vi "TPM with correction version 10-3-compare-1 scale factor.vi"() -> ()   [LabVIEW 2012]
uses:
  <vilib>/_Imagine Optic/VIs drivers/Data Haso/Wavefront parameters.ctl
  Program Files/Imagine Optic/Casao LabVIEW SDK/Casao/Casao/Loop prefs.ctl
  <vilib>/_Imagine Optic/VIs drivers/Data Haso/DataHaso.ctl
  <vilib>/Utility/file.llb/Read From Spreadsheet File (DBL).vi
  <vilib>/Utility/file.llb/Write To Spreadsheet File (DBL).vi
panel:
  in  "Scale factor":dbl=1.0
  out "output path":path
  out "Model Coefficients (µm) after":sgl[](array[numeric])
  out "Model Coefficients (µm) before":sgl[](array[numeric])
  in  "stop":bool
  out "Slice now":dbl
  in  "Iteration #":u16(ring)=1 items=["1"=1, "2"=2, "3"=3, "4"=4, "5"=5]
  in  "AoExp Time":dbl(ring)=0.5 items=["0.2s"=0.2, "0.5s"=0.5, "1.0s"=1.0, "1.5s"=1.5]
  out "after correction":T1
  in  "Filter y tilt":bool=TRUE
  in  "Filter x tilt":bool=TRUE
  in  "Curvature filter":bool=TRUE
  out "PV":dbl
  out "RMS":dbl
  in  "Matrix path":path=path "C:/Documents and Settings/User/Desktop/zw/20160128 1um bead command matrix.aomc"
  in  "Offset path":path=path "C:/Documents and Settings/User/Desktop/zw/2016-02-09 system resolution/100nm bead correction.dat"
  out "Camera image":u32[][](graph)
  out "RMS":dbl
  out "PV":dbl
  out "before correction":T1
  in  "Curvature filter":bool=TRUE
  in  "Filter y tilt":bool=TRUE
  in  "Filter x tilt":bool=TRUE
  out "after correction":dbl[][](graph) caption="Wavefront"
  out "before correction":dbl[][](graph) caption="Wavefront"
  in  "ImExp Time (s)":dbl(ring)=0.5 items=["0.2"=0.2, "0.5"=0.5, "1.0"=1.0, "4.0"=4.0, "8.0"=8.0]
  in  "Step size(um)":dbl
  in  "Laser Power%(0-100)":dbl=10.0
  in  "Slices #":dbl=1.0
  in  "Average Frame #":dbl=10.0
  in  "Correction":bool
  # "OFF"
  # "ON"
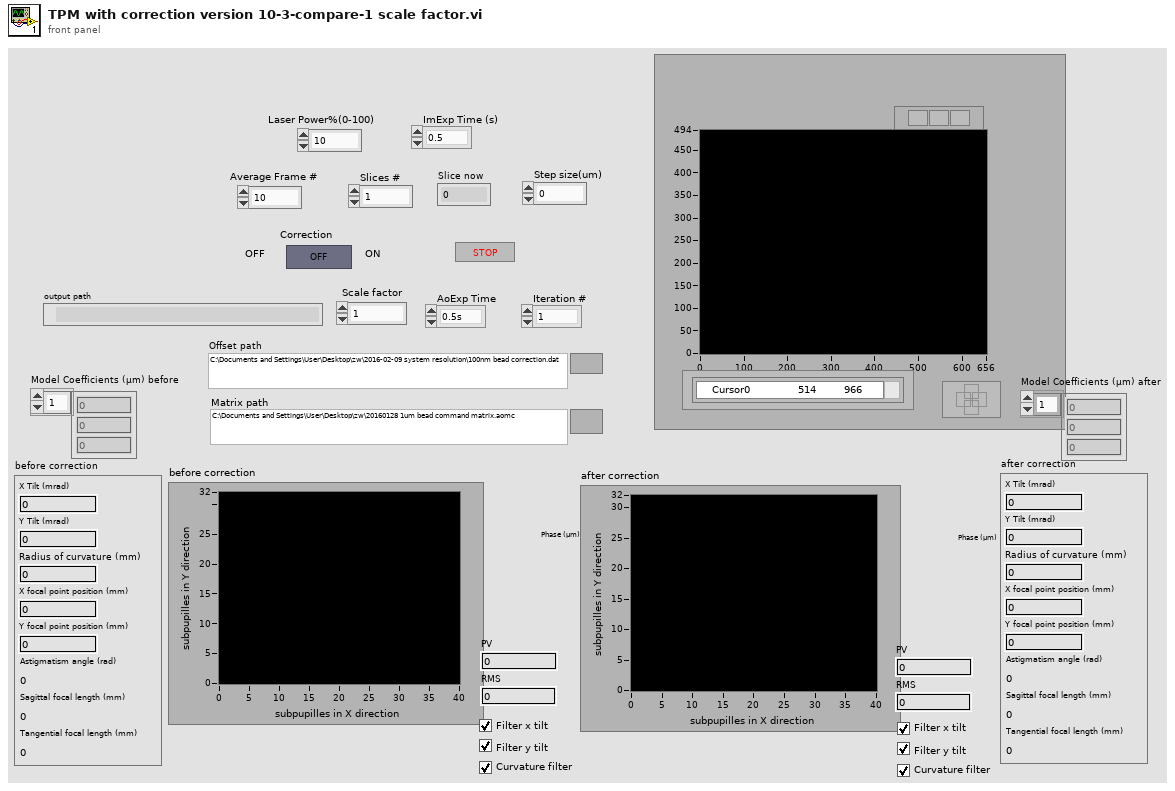
[diagram p1: front panel]
types:
  T1 = typedef "Wavefront parameters.ctl" = cluster{"X Tilt (mrad)":sgl, "Y Tilt (mrad)":sgl, "Radius of curvature (mm)":sgl, "X focal point position (mm)":sgl, "Y focal point position (mm)":sgl, "Astigmatism angle (rad)":sgl, "Sagittal focal length (mm)":sgl, "Tangential focal length (mm)":sgl}
  T2 = typedef "Loop prefs.ctl" = cluster{"Filter tilt on measurement (closed loop)":bool, "Correction gain (closed loop)":sgl, "Limit of subapertures off in CGP (%)":sgl, "Limit of saturated actuators (%)":sgl}
  T3 = cluster{"Filtre tilt X":bool, "Filtre tilt Y":bool, "Filtre courbure":bool}
  T4 = typedef "DataHaso.ctl" = i32
  T5 = cluster{"Measurement":T4, "Target":T4, "Manual target":T4}
  T6 = cluster{"Target for tilt":T4, "Target for focus":T4, "Target for all other aberrations":T4}
  T7 = typedef "Camera.ctl" = i32
  T8 = typedef "PhaseModul.ctl" = i32
  T9 = typedef "Haso.ctl" = i32
  T10 = typedef "Casao.ctl" = i32
  T11 = typedef "Image Compat.ctl" = cluster{"Signed/unsigned":bool, "Number of bits":T12, "Internal object id":i32, "Internal data id":i32}
  T12 = typedef "Data alignment enum.ctl" = enum16{"8", "16", "32"}
  T13 = typedef "Reconstruction prefs.ctl" = cluster{"Reconstruction type":enum16{"Modal", "Zonal"}, "Polynomial type":enum16{"Zernike", "Legendre"}, "Modal reconstruction prefs":T14, "Zonal reconstruction prefs":T17}
  T14 = typedef "Modal reconstruction prefs.ctl" = cluster{"Number of coefficients":u32, "Filtered coefficients":u32[], "RMS Zernike normalization":bool, "Matrix inversion method":u16, "Add zonal residual to modal fit ":bool, "Detection prefs":T15}
  T15 = typedef "PupilDetectionPrefs.ctl" = cluster{"Automatic pupil detection":bool, "Central occultation pupil":bool, "Semi-automatic pupil detection (find radius)":bool, "Semi-automatic pupil detection (find center)":bool, "Automatic pupil detection mode":enum16{"Contained", "Containing"}, "Start coordinates":cluster{"Pupil center (Zernike)":T16, "Pupil radius (Zernike)":sgl, "Pupil center (Legendre)":T16, "Pupil halfsize (Legendre)":T16}}
  T16 = typedef "Point2Df.ctl" = cluster{"X":sgl, "Y":sgl}
  T17 = typedef "Zonal reconstruction prefs.ctl" = cluster{"Number of weak iterations":u16, "Number of max iterations":u32, "Residual limit":sgl}
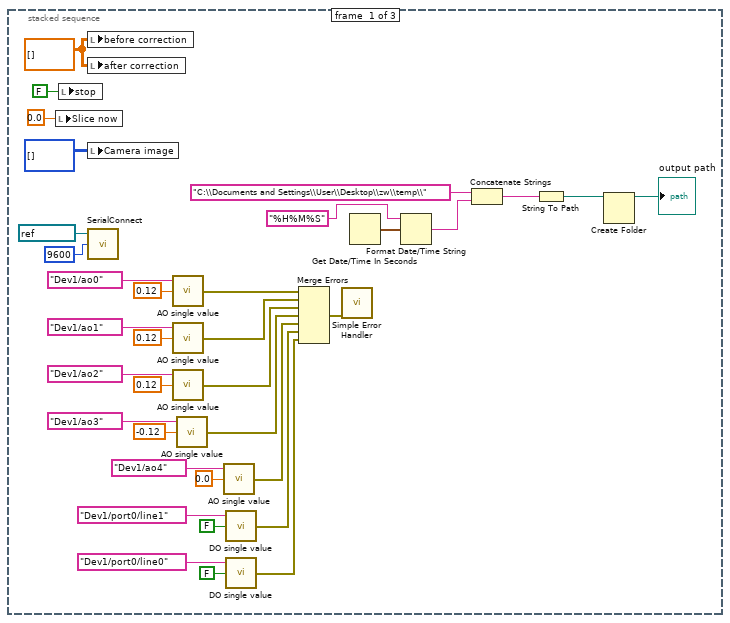
[diagram p2: hidden frame]
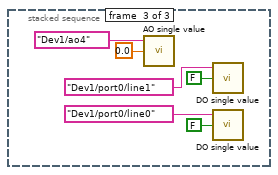
[diagram p11: hidden frame]
diagram:
  n1 = stacked-sequence {
    frame #0 {
      w34 = dbl[][] [] ("before correction")
      n2 = local write "Slice now"(0.0 ("Slice now")) -> ()
      n3 = local write "stop"(FALSE ("stop")) -> ()
      n4 = local write "before correction"(w34) -> ()
      n5 = local write "after correction"(w34) -> ()
      n6 = local write "Camera image"(u32[][] [] ("Camera image")) -> ()
      n7 = call "SerialConnect.vi"("baud rate (9600)"=u32 9600, "VISA resource name"=refnum<visa-resource-name> "COM1") -> ()  [unwired: 1 in, 3 out]
      n8 = call "AO single value.vi"("data"=0.12, "physical channels"=tag "Dev1/ao0") -> ("error out"=w17:errorcluster)  [unwired: 1 in]
      n9 = call "AO single value.vi"("data"=0.12, "physical channels"=tag "Dev1/ao1") -> ("error out"=w16:errorcluster)  [unwired: 1 in]
      n10 = call "AO single value.vi"("data"=0.12, "physical channels"=tag "Dev1/ao2") -> ("error out"=w15:errorcluster)  [unwired: 1 in]
      n11 = call "AO single value.vi"("data"=-0.12, "physical channels"=tag "Dev1/ao3") -> ("error out"=w14:errorcluster)  [unwired: 1 in]
      n12 = call "AO single value.vi"("data"=0.0, "physical channels"=tag "Dev1/ao4") -> ("error out"=w13:errorcluster)  [unwired: 1 in]
      n13 = call "DO single value.vi"("data"=FALSE, "lines"=tag "Dev1/port0/line1") -> ("error out"=w12:errorcluster)  [unwired: 1 in]
      n14 = call "DO single value.vi"("data"=FALSE, "lines"=tag "Dev1/port0/line0") -> ("error out"=w10:errorcluster)  [unwired: 1 in]
      n15 = Merge Errors(w17, w16, w15, w14, w13, w12, w10) -> (w11:errorcluster)
      n16 = call <vilib>:"Simple Error Handler.vi"("error in (no error)"=w11) -> ()  [unwired: 4 in, 5 out]
      n17 = Get Date/Time In Seconds() -> (seconds since 1Jan1904=w7:timestamp)
      n18 = Format Date/Time String(time format string (%c)="%H%M%S", seconds (now)=w7) -> (date/time string=w4:string)  [unwired: 1 in]
      n19 = Concatenate Strings("C:\\Documents and Settings\\User\\Desktop\\zw\\temp\\" ("string"), w4) -> (w3:string)
      n20 = String To Path(string=w3) -> (path=w2:path)
      n21 = Create Folder(path (use dialog)=w2) -> (created path=→"output path":path)  [unwired: 2 in, 2 out]
    }
    frame #1 {
      n22 = case shown="False" "Correction" {
        frame False {
          n23 = flat-sequence {
            frame #0 {
              n24 = call "AO single value.vi"("data"=-5.0, "physical channels"=tag "Dev1/ao5") -> ()  [unwired: 1 in, 1 out]
              n25 = call "DO single value.vi"("data"=TRUE, "lines"=tag "Dev1/port0/line1") -> ()  [unwired: 1 in, 1 out]
              n26 = call "DO single value.vi"("data"=FALSE, "lines"=tag "Dev1/port0/line0") -> ()  [unwired: 1 in, 1 out]
            }
            frame #1 {
              n27 = for {
                N: "Slices #" -> [_]
                i -> [w47]
                n28 = local read "stop"() -> (w45:bool)
                n29 = Not(x=w45) -> (.not. x?=w44:bool)
                n30 = Increment(x=w47) -> (x+1=w46:i32)
                n31 = case shown="True" w44 {
                  tunnel: w46 -> [_ w48]
                  frame False {
                  }
                  frame True {
                    n32 = flat-sequence {
                      frame #0 {
                        n33 = for {
                          N: "Average Frame #" -> [_]
                          n34 = local read "stop"() -> (w50:bool)
                          n35 = Not(x=w50) -> (.not. x?=w51:bool)
                          n36 = case shown="True" w51 {
                            frame False {
                            }
                            frame True {
                              n37 = flat-sequence {
                                tunnel: [w53] -> w52
                                tunnel: w52 -> [w75]
                                frame #0 {
                                n38 = local read "Laser Power%(0-100)"() -> (w64:dbl)
                                n39 = local read "ImExp Time (s)"() -> (w63:dbl)
                                n40 = call "waveform gen.vi"("Boolean"=TRUE, "Exposure Time (s)"=w63, "Laser Power%(0-100)"=w64) -> ("waveform"=w61:waveform(dbl)[])
                                n41 = Index Array(array=w61, index=4) -> (element=w62:waveform(dbl))
                                n42 = call "AO triggle.vi"("physical channels"=tag "Dev1/ao0:4", "data"=w61, "waveform"=w62, "trig source"=tag "/Dev1/PFI1") -> ("task out"=w58:refnum<k21>, "error out"=w55:errorcluster)  [unwired: 1 in]
                                n43 = call "DO single value.vi"("error in"=w55, "data"=TRUE, "lines"=tag "Dev1/port0/line0") -> ("error out"=w54:errorcluster)
                                n44 = while {
                                tunnel: [w73] -> w67
                                tunnel: [w72] -> w66
                                tunnel: w58 -> [w70]
                                tunnel: w54 -> [w69]
                                stop <- w71 stop-if-true
                                n45 = call <vilib>:"DAQmx Is Task Done.vi"("task/channels in"=w70, "error in"=w69) -> ("task out"=w73:refnum<k21>, "task done?"=w71:bool, "error out"=w72:errorcluster)  [unwired: 11 in]
                                }
                                n46 = call <vilib>:"DAQmx Clear Task.vi"("task in"=w67, "error in"=w66) -> ("error out"=w53:errorcluster)  [unwired: 13 in]
                                }
                                frame #1 {
                                n47 = call "DO single value.vi"("error in"=w75, "data"=FALSE, "lines"=tag "Dev1/port0/line0") -> ("error out"=w74:errorcluster)
                                n48 = call "AO single value.vi"("error in"=w74, "data"=0.0, "physical channels"=tag "Dev1/ao4") -> ()  [unwired: 1 out]
                                }
                              }
                            }
                          }
                        }
                      }
                      frame #1 {
                        n49 = local read "Step size(um)"() -> (w80:dbl)
                        n50 = Multiply(x=w80, y=10.0) -> (x*y=w82:dbl)
                        n51 = Number To Decimal String(number=w82) -> (decimal integer string=w85:string)  [unwired: 1 in]
                        n52 = Concatenate Strings("movrel z=", w85) -> (w84:string)
                        n53 = call "WriteCmd.vi"("Command"=w84, "VISA resource name"=refnum<visa-resource-name> "COM1") -> ()  [unwired: 1 in, 1 out]
                      }
                      frame #2 {
                        n54 = Wait (ms)(milliseconds to wait=u32 100) -> ()  [unwired: 1 out]
                      }
                    }
                    n55 = local write "Slice now"(w48) -> ()
                  }
                }
              }
            }
            frame #2 {
            }
          }
        }
        frame True {
          n56 = flat-sequence {
            tunnel: [w103] -> w95
            tunnel: [w105] -> w94
            tunnel: [w104] -> w93
            tunnel: [w103] -> w92
            tunnel: [w102] -> w91
            tunnel: [w101] -> w89
            tunnel: [w96] -> w88
            tunnel: w95 -> [w122]
            tunnel: w94 -> [w121]
            tunnel: w93 -> [w120]
            tunnel: w92 -> [w116]
            tunnel: w91 -> [w114]
            tunnel: [w119] -> w90
            tunnel: w89 -> [w118]
            tunnel: w88 -> [w112]
            tunnel: w90 -> [w646]
            frame #0 {
              n57 = call "AO single value.vi"("data"=0.0, "physical channels"=tag "Dev1/ao4") -> ()  [unwired: 1 in, 1 out]
              n58 = local read "AoExp Time"() -> (w106:dbl)
              n59 = call-poly <vilib>:"Read From Spreadsheet File.vi"("format (%.3f)"="%.8f", "file path (dialog if empty)"="Offset path") -> ("first row"=w96:dbl[])  [unwired: 5 in, 4 out]
              n60 = call "DO single value.vi"("data"=TRUE, "lines"=tag "Dev1/port0/line1") -> ()  [unwired: 1 in, 1 out]
              n61 = call "DO single value.vi"("data"=FALSE, "lines"=tag "Dev1/port0/line0") -> ()  [unwired: 1 in, 1 out]
              n62 = call "AO init.vi"("Exposure duration specified (s)"=w106, "Commands in"=w96, "Matrix path"="Matrix path") -> ("error out"=w103:errorcluster, "Camera"=w105:T7, "Mirror"=w101:T8, "Haso"=w104:T9, "Casao"=w102:T10)  [unwired: 3 in, 1 out]
            }
            frame #1 {
              n63 = local read "Slices #"() -> (w123:dbl)
              n64 = call "Casao Set Preferences.vi"("error in (no error)"=w116, "Loop preferences"=T2 {"Filter tilt on measurement (closed loop)"=FALSE, "Correction gain (closed loop)"=0.75, "Limit of subapertures off in CGP (%)"=0.0, "Limit of saturated actuators (%)"=0.0}, "Casao"=w114) -> ("error out"=w115:errorcluster, "Casao (dup)"=w113:T10)  [unwired: 3 in]
              n65 = for {
                N: w123 -> [_]
                tunnel: w122 -> [w139]
                tunnel: w121 -> [w138]
                tunnel: w120 -> [w137]
                tunnel: w115 -> [w125]
                tunnel: [w136] -> w119
                tunnel: w118 -> [w127]
                tunnel: w113 -> [w135]
                tunnel: w112 -> [w128]
                i -> [w131]
                n66 = local read "stop"() -> (w133:bool)
                n67 = call "PhaseModul apply command.vi"("error in (no error)"=w125, "Commands in"=w128, "Mirror"=w127) -> ("error out"=w124:errorcluster, "Mirror (dup)"=w126:T8)  [unwired: 2 in, 1 out]
                n68 = Increment(x=w131) -> (x+1=w134:i32)
                n69 = local write "Slice now"(w134) -> ()
                n70 = Not(x=w133) -> (.not. x?=w132:bool)
                n71 = case shown="True" w132 {
                  tunnel: w139 -> [_ w174]
                  tunnel: w138 -> [_ w173]
                  tunnel: w137 -> [_ w172]
                  tunnel: w124 -> [_ w171]
                  tunnel: [w140 w168] -> w136
                  tunnel: w126 -> [_ w170]
                  tunnel: w135 -> [w140 w169]
                  frame False {
                  }
                  frame True {
                    n72 = flat-sequence {
                      tunnel: w169 -> [w179]
                      tunnel: w170 -> [w180]
                      tunnel: w171 -> [w181]
                      tunnel: w172 -> [w182]
                      tunnel: w173 -> [w183]
                      tunnel: w174 -> [w184]
                      tunnel: [w184] -> w146
                      tunnel: [w183] -> w145
                      tunnel: [w182] -> w144
                      tunnel: [w181] -> w143
                      tunnel: [w180] -> w142
                      tunnel: [w179] -> w141
                      tunnel: [w218] -> w167
                      tunnel: [w217] -> w166
                      tunnel: [w216] -> w165
                      tunnel: [w211] -> w164
                      tunnel: [w212] -> w163
                      tunnel: [w213] -> w162
                      tunnel: w146 -> [w218]
                      tunnel: w145 -> [w217]
                      tunnel: w144 -> [w216]
                      tunnel: w143 -> [w212]
                      tunnel: w142 -> [w213]
                      tunnel: w141 -> [w211]
                      tunnel: w167 -> [w260]
                      tunnel: w166 -> [w259]
                      tunnel: w165 -> [w258]
                      tunnel: w164 -> [w257]
                      tunnel: w163 -> [w256]
                      tunnel: [w236] -> w161
                      tunnel: [w235] -> w160
                      tunnel: [w231] -> w159
                      tunnel: [w229] -> w158
                      tunnel: [w227] -> w157
                      tunnel: w162 -> [w222]
                      tunnel: [w221] -> w156
                      tunnel: [w219] -> w155
                      tunnel: w161 -> [w402]
                      tunnel: w160 -> [w401]
                      tunnel: w159 -> [w399]
                      tunnel: w158 -> [w398]
                      tunnel: w157 -> [w397]
                      tunnel: [w396] -> w154
                      tunnel: w156 -> [w395]
                      tunnel: [w394] -> w153
                      tunnel: [w393] -> w152
                      tunnel: [w392] -> w151
                      tunnel: [w391] -> w150
                      tunnel: [w390] -> w149
                      tunnel: w155 -> [w389]
                      tunnel: [w389] -> w148
                      tunnel: w154 -> [w609]
                      tunnel: [w609] -> w147
                      tunnel: w153 -> [w599]
                      tunnel: w152 -> [w598]
                      tunnel: w151 -> [w597]
                      tunnel: w150 -> [w587]
                      tunnel: w149 -> [w588]
                      tunnel: w148 -> [w586]
                      tunnel: w147 -> [w610]
                      tunnel: [w610] -> w168
                      frame #0 {
                        n73 = Wait (ms)(milliseconds to wait=u32 100) -> ()  [unwired: 1 out]
                        n74 = local read "Average Frame #"() -> (w178:dbl)
                        n75 = call "AO single value.vi"("data"=-5.0, "physical channels"=tag "Dev1/ao5") -> ()  [unwired: 1 in, 1 out]
                        n76 = for {
                          N: w178 -> [_]
                          n77 = local read "stop"() -> (w185:bool)
                          n78 = Not(x=w185) -> (.not. x?=w186:bool)
                          n79 = case shown="True" w186 {
                            frame False {
                            }
                            frame True {
                              n80 = flat-sequence {
                                frame #0 {
                                n81 = local read "Laser Power%(0-100)"() -> (w197:dbl)
                                n82 = local read "ImExp Time (s)"() -> (w196:dbl)
                                n83 = call "waveform gen.vi"("Boolean"=TRUE, "Exposure Time (s)"=w196, "Laser Power%(0-100)"=w197) -> ("waveform"=w194:waveform(dbl)[])
                                n84 = Index Array(array=w194, index=4) -> (element=w195:waveform(dbl))
                                n85 = call "AO triggle.vi"("physical channels"=tag "Dev1/ao0:4", "data"=w194, "waveform"=w195, "trig source"=tag "/Dev1/PFI0") -> ("task out"=w191:refnum<k21>, "error out"=w188:errorcluster)  [unwired: 1 in]
                                n86 = call "DO single value.vi"("error in"=w188, "data"=TRUE, "lines"=tag "Dev1/port0/line0") -> ("error out"=w187:errorcluster)
                                n87 = while {
                                tunnel: [w206] -> w200
                                tunnel: [w205] -> w199
                                tunnel: w191 -> [w203]
                                tunnel: w187 -> [w202]
                                stop <- w204 stop-if-true
                                n88 = call <vilib>:"DAQmx Is Task Done.vi"("task/channels in"=w203, "error in"=w202) -> ("task out"=w206:refnum<k21>, "task done?"=w204:bool, "error out"=w205:errorcluster)  [unwired: 11 in]
                                }
                                n89 = call <vilib>:"DAQmx Clear Task.vi"("task in"=w200, "error in"=w199) -> ()  [unwired: 13 in, 1 out]
                                }
                                frame #1 {
                                n90 = call "AO single value.vi"("data"=0.0, "physical channels"=tag "Dev1/ao4") -> ()  [unwired: 1 in, 1 out]
                                n91 = call "DO single value.vi"("data"=FALSE, "lines"=tag "Dev1/port0/line0") -> ()  [unwired: 1 in, 1 out]
                                }
                              }
                            }
                          }
                        }
                      }
                      frame #1 {
                        n92 = call "AO single value.vi"("data"=1.0, "physical channels"=tag "Dev1/ao5") -> ()  [unwired: 1 in, 1 out]
                      }
                      frame #2 {
                        n93 = flat-sequence {
                          tunnel: [w269] -> w255
                          tunnel: [w268] -> w254
                          tunnel: [w267] -> w253
                          tunnel: [w266] -> w252
                          tunnel: [w265] -> w251
                          tunnel: w258 -> [w267]
                          tunnel: w259 -> [w268]
                          tunnel: w260 -> [w269]
                          tunnel: [w264] -> w250
                          tunnel: w257 -> [w264]
                          tunnel: [w263] -> w249
                          tunnel: w256 -> [w263]
                          tunnel: [w262] -> w223
                          tunnel: w222 -> [w262]
                          tunnel: w255 -> [w285]
                          tunnel: w254 -> [w286]
                          tunnel: w253 -> [w287]
                          tunnel: [w287] -> w248
                          tunnel: [w284] -> w247
                          tunnel: [w283] -> w246
                          tunnel: [w282] -> w245
                          tunnel: w252 -> [w282]
                          tunnel: [w281] -> w244
                          tunnel: w251 -> [w281]
                          tunnel: [w280] -> w243
                          tunnel: w250 -> [w280]
                          tunnel: [w279] -> w242
                          tunnel: w249 -> [w279]
                          tunnel: [w278] -> w224
                          tunnel: w223 -> [w278]
                          tunnel: w248 -> [w299]
                          tunnel: [w299] -> w239
                          tunnel: [w298] -> w240
                          tunnel: w247 -> [w298]
                          tunnel: [w297] -> w241
                          tunnel: w246 -> [w297]
                          tunnel: w245 -> [w292]
                          tunnel: w244 -> [w291]
                          tunnel: [w290] -> w238
                          tunnel: w243 -> [w290]
                          tunnel: [w289] -> w237
                          tunnel: w242 -> [w289]
                          tunnel: [w288] -> w225
                          tunnel: w224 -> [w288]
                          tunnel: w241 -> [w381]
                          tunnel: w240 -> [w341]
                          tunnel: w239 -> [w342]
                          tunnel: w238 -> [w367]
                          tunnel: w237 -> [w366]
                          tunnel: [w345] -> w234
                          tunnel: [w344] -> w233
                          tunnel: [w343] -> w232
                          tunnel: [w342] -> w230
                          tunnel: [w341] -> w228
                          tunnel: [w340] -> w226
                          tunnel: w225 -> [w339]
                          tunnel: [w339] -> w220
                          tunnel: [w313] -> w219
                          tunnel: [w387] -> w235
                          tunnel: [w388] -> w236
                          tunnel: w234 -> [w388]
                          tunnel: w233 -> [w387]
                          tunnel: w232 -> [w386]
                          tunnel: [w385] -> w231
                          tunnel: w230 -> [w385]
                          tunnel: [w384] -> w229
                          tunnel: w228 -> [w384]
                          tunnel: [w383] -> w227
                          tunnel: w226 -> [w383]
                          tunnel: [w382] -> w221
                          tunnel: w220 -> [w382]
                          frame #0 {
                            n94 = local read "Laser Power%(0-100)"() -> (w275:dbl)
                            n95 = local read "AoExp Time"() -> (w274:dbl)
                            n96 = local read "Scale factor"() -> (w261:dbl)
                            n97 = call "waveform gen_scale factor.vi"("Scale factor"=w261, "Boolean"=FALSE, "Exposure Time (s)"=w274, "Laser Power%(0-100)"=w275) -> ("waveform"=w273:waveform(dbl)[])
                            n98 = Index Array(array=w273, index=4) -> (element=w272:waveform(dbl))
                            n99 = call "AO triggle.vi"("physical channels"=tag "Dev1/ao0:4", "data"=w273, "waveform"=w272, "trig source"=tag "/Dev1/PFI1") -> ("task out"=w266:refnum<k21>, "error out"=w265:errorcluster)  [unwired: 1 in]
                          }
                          frame #1 {
                            n100 = call <vilib>:"Camera Start.vi"("error in (no error)"=w285, "camera"=w286) -> ("error out"=w283:errorcluster, "camera (dup)"=w284:T7)  [unwired: 4 in]
                          }
                          frame #2 {
                            n101 = while {
                              tunnel: [w304] -> w294
                              tunnel: [w303] -> w293
                              tunnel: w292 -> [w301]
                              tunnel: w291 -> [w300]
                              stop <- w302 stop-if-true
                              n102 = call <vilib>:"DAQmx Is Task Done.vi"("task/channels in"=w301, "error in"=w300) -> ("task out"=w304:refnum<k21>, "task done?"=w302:bool, "error out"=w303:errorcluster)  [unwired: 11 in]
                            }
                            n103 = call "DO single value.vi"("data"=TRUE, "lines"=tag "Dev1/port0/line0") -> ()  [unwired: 1 in, 1 out]
                            n104 = call <vilib>:"DAQmx Clear Task.vi"("task in"=w294, "error in"=w293) -> ()  [unwired: 13 in, 1 out]
                          }
                          frame #3 {
                            n105 = call <vilib>:"Camera Get image.vi"("error in (no error)"=w381, "camera"=w341) -> ("error out"=w363:errorcluster, "Image"=w364:T11, "camera (dup)"=w365:T7)  [unwired: 3 in]
                            n106 = call <vilib>:"Camera Stop.vi"("error in (no error)"=w363, "camera"=w365) -> ()  [unwired: 4 in, 2 out]
                            n107 = call "Image get data.vi"("error in (no error)"=w363, "Image Compat"=w364) -> ("error out"=w353:errorcluster, "Array"=w362:u32[][], "Image Compat (dup)"=w352:T11)  [unwired: 3 in]
                            n108 = call "AO single value.vi"("data"=0.0, "physical channels"=tag "Dev1/ao4") -> ()  [unwired: 1 in, 1 out]
                            n109 = local write "Camera image"(w362) -> ()
                            n110 = call <vilib>:"Haso compute slopes.vi"("error in (no error)"=w353, "Image Compat"=w352, "Haso"=w342) -> ("error out"=w311:errorcluster, "Data Haso"=w315:T4)  [unwired: 1 in, 2 out]
                            n111 = call "DO single value.vi"("data"=FALSE, "lines"=tag "Dev1/port0/line0") -> ()  [unwired: 1 in, 1 out]
                            n112 = call "DataHaso ctor copie.vi"("error in (no error)"=w311, "DataHaso"=w315) -> ("error out"=w310:errorcluster, "new DataHaso"=w313:T4, "DataHaso (dup)"=w312:T4)  [unwired: 3 in]
                            n113 = call "DataHaso get reconstruction prefs.vi"("error in (no error)"=w310, "Data Haso"=w312) -> ("error out"=w326:errorcluster, "Reconstruction Preferences"=w322:T13, "Data Haso (dup)"=w325:T4)  [unwired: 3 in]
                            n114 = Bundle By Name(cluster=w322, "Reconstruction type"=enum16{"Modal", "Zonal"}."Modal", "Polynomial type"=enum16{"Zernike", "Legendre"}."Zernike", "Modal reconstruction prefs.Number of coefficients"=u32 32) -> (w321:T13)
                            n115 = call <vilib>:"DataHaso set reconstruction prefs.vi"("error in (no error)"=w326, "Reconstruction Preferences"=w321, "Data Haso"=w325) -> ("error out"=w323:errorcluster, "Data Haso (dup)"=w324:T4)  [unwired: 3 in]
                            n116 = call "DataHaso get modal coefficients.vi"("error in (no error)"=w323, "Data Haso"=w324) -> ("error out"=w316:errorcluster, "Coefficients (µm)"=w327:sgl[], "Data Haso (dup)"=w317:T4)  [unwired: 3 in]
                            "Model Coefficients (µm) before" <- w327
                            n117 = Bundle By Name(cluster=T3 {"Filtre tilt X"=FALSE, "Filtre tilt Y"=FALSE, "Filtre courbure"=FALSE} ("Filtre"), "Filtre tilt X"="Filter x tilt", "Filtre tilt Y"="Filter y tilt", "Filtre courbure"="Curvature filter") -> (w347:T3)
                            n118 = call <vilib>:"DataHaso parameters.vi"("error in (no error)"=w316, "Data Haso"=w317) -> ("error out"=w360:errorcluster, "Parameters"=w335:T1, "Data Haso (dup)"=w361:T4)  [unwired: 3 in]
                            "before correction" <- w335
                            n119 = control-ref of="before correction"() -> (w346:refnum<vi>)
                            n120 = Cluster To Array(cluster=w335) -> (array=w336:sgl[])
                            n121 = call "DataHaso filter tilt or curvature.vi"("error in (no error)"=w360, "Filter (default: all true)"=w347, "Data Haso"=w361) -> ("error out"=w358:errorcluster, "Data Haso (dup)"=w359:T4)  [unwired: 3 in]
                            n122 = local read "Slice now"() -> (w329:dbl)
                            n123 = call "DataHaso phase.vi"("error in (no error)"=w358, "Data Haso"=w359) -> ("error out"=w356:errorcluster, "Phase (µm)"=w357:i32, "Data Haso (dup)"=w314:T4)  [unwired: 3 in]
                            n124 = Number To Decimal String(number=w329) -> (decimal integer string=w331:string)  [unwired: 1 in]
                            n125 = call "Formatter Intensity Graph.vi"("error in (no error)"=w356, "Intensity Graph"=w346, "Surface with pupil"=w357) -> ("error out"=w354:errorcluster, "Surface with pupil (dup)"=w355:i32)  [unwired: 2 in, 1 out]
                            n126 = call <vilib>:"Surface with pupil get stats.vi"("error in (no error)"=w354, "Surface Avec Pupille"=w355) -> ("error out"=w340:errorcluster, "PV"=w338:sgl, "RMS"=w337:dbl)  [unwired: 2 in, 1 out]
                            "PV" <- w338
                            "RMS" <- w337
                            n127 = local read "output path"() -> (w307:path)
                            n128 = Concatenate Strings("before_slice", w331, ".dat") -> (w306:string)
                            n129 = Build Path(base path=w307, name or relative path=w306) -> (appended path=w305:path)
                            n130 = Build Array (concatenate)(w338, w337, w336, w327) -> (w334:dbl[])
                            n131 = Merge Errors(w340, w366) -> (w376:errorcluster)
                            n132 = Bundle By Name(cluster=T6 {"Target for tilt"=0, "Target for focus"=0, "Target for all other aberrations"=0} ("References"), "Target for tilt"=w313, "Target for focus"=w313) -> (w379:T6)
                            n133 = call "DataHaso ctor copie.vi"("error in (no error)"=w376, "DataHaso"=w314) -> ("error out"=w378:errorcluster, "new DataHaso"=w377:T4)  [unwired: 3 in, 1 out]
                            n134 = call-poly <vilib>:"Write To Spreadsheet File.vi"("transpose? (no:F)"=TRUE, "format (%.3f)"="%.6f", "1D data"=w334, "file path (dialog if empty)"=w305) -> ()  [unwired: 4 in, 1 out]
                            n135 = call "Casao Compute target.vi"("error in (no error)"=w378, "Targets"=w379, "DataHaso"=w377, "Casao"=w367) -> ("error out"=w374:errorcluster, "DataHaso (dup)"=w343:T4, "Casao (dup)"=w375:T10)  [unwired: 1 out]
                            n136 = Bundle By Name(cluster=T5 {"Measurement"=0, "Target"=0, "Manual target"=0} ("Slopes"), "Measurement"=w314, "Target"=w343) -> (w373:T5)
                            n137 = call "Casao get correction commands.vi"("Casao"=w375, "Slopes"=w373, "error in (no error)"=w374) -> ("Casao (dup)"=w345:T10, "Commands"=w370:sgl[], "error out"=w371:errorcluster)  [unwired: 2 in, 2 out]
                            n138 = call "PhaseModul apply command.vi"("error in (no error)"=w371, "Commands in"=w370, "Mirror"=w339) -> ("error out"=w344:errorcluster)  [unwired: 2 in, 2 out]
                          }
                          frame #4 {
                            n139 = call "DataHaso dtor.vi"("Data Haso"=w386) -> ()  [unwired: 6 in, 1 out]
                          }
                        }
                      }
                      frame #3 {
                        n140 = for {
                          N: "Iteration #" -> [_]
                          tunnel: w402 -> [w431]
                          tunnel: w401 -> [w430]
                          tunnel: w399 -> [w429]
                          tunnel: w398 -> [w428]
                          tunnel: w397 -> [w427]
                          tunnel: [w425] -> w396
                          tunnel: w395 -> [w420]
                          tunnel: [w419] -> w394
                          tunnel: [w417] -> w393
                          tunnel: [w415] -> w392
                          tunnel: [w413] -> w391
                          tunnel: [w410] -> w390
                          tunnel: w389 -> [w409]
                          i -> [w408]
                          n141 = Increment(x=w408) -> (x+1=w407:i32)
                          n142 = flat-sequence {
                            tunnel: [w456] -> w450
                            tunnel: [w457] -> w449
                            tunnel: [w458] -> w448
                            tunnel: [w462] -> w447
                            tunnel: [w461] -> w446
                            tunnel: [w460] -> w445
                            tunnel: [w459] -> w444
                            tunnel: w431 -> [w460]
                            tunnel: w430 -> [w459]
                            tunnel: w429 -> [w458]
                            tunnel: w428 -> [w457]
                            tunnel: w427 -> [w456]
                            tunnel: [w455] -> w421
                            tunnel: w420 -> [w455]
                            tunnel: w407 -> [w453]
                            tunnel: [w452] -> w404
                            tunnel: w450 -> [w479]
                            tunnel: w449 -> [w480]
                            tunnel: w448 -> [w481]
                            tunnel: [w481] -> w443
                            tunnel: [w478] -> w442
                            tunnel: [w477] -> w441
                            tunnel: [w476] -> w440
                            tunnel: w447 -> [w476]
                            tunnel: [w475] -> w439
                            tunnel: w446 -> [w475]
                            tunnel: [w474] -> w438
                            tunnel: w445 -> [w474]
                            tunnel: [w473] -> w437
                            tunnel: w444 -> [w473]
                            tunnel: [w472] -> w422
                            tunnel: w421 -> [w472]
                            tunnel: [w471] -> w405
                            tunnel: w404 -> [w471]
                            tunnel: w443 -> [w494]
                            tunnel: [w494] -> w434
                            tunnel: [w493] -> w435
                            tunnel: w442 -> [w493]
                            tunnel: [w492] -> w436
                            tunnel: w441 -> [w492]
                            tunnel: w440 -> [w487]
                            tunnel: w439 -> [w486]
                            tunnel: [w485] -> w433
                            tunnel: w438 -> [w485]
                            tunnel: [w484] -> w432
                            tunnel: w437 -> [w484]
                            tunnel: [w483] -> w423
                            tunnel: w422 -> [w483]
                            tunnel: [w482] -> w406
                            tunnel: w405 -> [w482]
                            tunnel: w436 -> [w562]
                            tunnel: w435 -> [w563]
                            tunnel: w434 -> [w564]
                            tunnel: w433 -> [w549]
                            tunnel: w432 -> [w548]
                            tunnel: [w528] -> w426
                            tunnel: [w527] -> w424
                            tunnel: w423 -> [w507]
                            tunnel: [w523] -> w418
                            tunnel: [w522] -> w416
                            tunnel: [w521] -> w414
                            tunnel: [w520] -> w412
                            tunnel: [w509] -> w411
                            tunnel: w409 -> [w506]
                            tunnel: w406 -> [w503]
                            tunnel: [w500] -> w403
                            tunnel: w426 -> [w576]
                            tunnel: [w575] -> w425
                            tunnel: w424 -> [w575]
                            tunnel: [w574] -> w419
                            tunnel: w418 -> [w574]
                            tunnel: [w573] -> w417
                            tunnel: w416 -> [w573]
                            tunnel: [w572] -> w415
                            tunnel: w414 -> [w572]
                            tunnel: [w568] -> w413
                            tunnel: w412 -> [w569]
                            tunnel: w411 -> [w571]
                            tunnel: [w571] -> w410
                            tunnel: w403 -> [w570]
                            frame #0 {
                              n143 = local read "Laser Power%(0-100)"() -> (w468:dbl)
                              n144 = local read "AoExp Time"() -> (w467:dbl)
                              n145 = local read "Scale factor"() -> (w451:dbl)
                              n146 = call "waveform gen_scale factor.vi"("Scale factor"=w451, "Boolean"=FALSE, "Exposure Time (s)"=w467, "Laser Power%(0-100)"=w468) -> ("waveform"=w466:waveform(dbl)[])
                              n147 = local read "Iteration #"() -> (w454:u16)
                              n148 = Index Array(array=w466, index=4) -> (element=w465:waveform(dbl))
                              n149 = Less?(x=w454, y=w453) -> (x < y?=w452:bool)
                              n150 = call "AO triggle.vi"("physical channels"=tag "Dev1/ao0:4", "data"=w466, "waveform"=w465, "trig source"=tag "/Dev1/PFI1") -> ("task out"=w462:refnum<k21>, "error out"=w461:errorcluster)  [unwired: 1 in]
                            }
                            frame #1 {
                              n151 = call <vilib>:"Camera Start.vi"("error in (no error)"=w479, "camera"=w480) -> ("error out"=w477:errorcluster, "camera (dup)"=w478:T7)  [unwired: 4 in]
                            }
                            frame #2 {
                              n152 = while {
                                tunnel: [w499] -> w489
                                tunnel: [w498] -> w488
                                tunnel: w487 -> [w496]
                                tunnel: w486 -> [w495]
                                stop <- w497 stop-if-true
                                n153 = call <vilib>:"DAQmx Is Task Done.vi"("task/channels in"=w496, "error in"=w495) -> ("task out"=w499:refnum<k21>, "task done?"=w497:bool, "error out"=w498:errorcluster)  [unwired: 11 in]
                              }
                              n154 = call "DO single value.vi"("data"=TRUE, "lines"=tag "Dev1/port0/line0") -> ()  [unwired: 1 in, 1 out]
                              n155 = call <vilib>:"DAQmx Clear Task.vi"("task in"=w489, "error in"=w488) -> ()  [unwired: 13 in, 1 out]
                            }
                            frame #3 {
                              n156 = call <vilib>:"Camera Get image.vi"("error in (no error)"=w562, "camera"=w563) -> ("error out"=w545:errorcluster, "Image"=w546:T11, "camera (dup)"=w547:T7)  [unwired: 3 in]
                              n157 = call <vilib>:"Camera Stop.vi"("error in (no error)"=w545, "camera"=w547) -> ()  [unwired: 4 in, 2 out]
                              n158 = call "Image get data.vi"("error in (no error)"=w545, "Image Compat"=w546) -> ("error out"=w535:errorcluster, "Array"=w544:u32[][], "Image Compat (dup)"=w534:T11)  [unwired: 3 in]
                              n159 = call "AO single value.vi"("data"=0.0, "physical channels"=tag "Dev1/ao4") -> ()  [unwired: 1 in, 1 out]
                              n160 = local write "Camera image"(w544) -> ()
                              n161 = call <vilib>:"Haso compute slopes.vi"("error in (no error)"=w535, "Image Compat"=w534, "Haso"=w564) -> ("error out"=w512:errorcluster, "Data Haso"=w511:T4)  [unwired: 1 in, 2 out]
                              n162 = call "DO single value.vi"("data"=FALSE, "lines"=tag "Dev1/port0/line0") -> ()  [unwired: 1 in, 1 out]
                              n163 = call "DataHaso get reconstruction prefs.vi"("error in (no error)"=w512, "Data Haso"=w511) -> ("error out"=w518:errorcluster, "Reconstruction Preferences"=w517:T13, "Data Haso (dup)"=w519:T4)  [unwired: 3 in]
                              n164 = Bundle By Name(cluster=w517, "Reconstruction type"=enum16{"Modal", "Zonal"}."Modal", "Polynomial type"=enum16{"Zernike", "Legendre"}."Zernike", "Modal reconstruction prefs.Number of coefficients"=u32 32) -> (w516:T13)
                              n165 = call <vilib>:"DataHaso set reconstruction prefs.vi"("error in (no error)"=w518, "Reconstruction Preferences"=w516, "Data Haso"=w519) -> ("error out"=w504:errorcluster, "Data Haso (dup)"=w505:T4)  [unwired: 3 in]
                              n166 = call "DataHaso get modal coefficients.vi"("error in (no error)"=w504, "Data Haso"=w505) -> ("error out"=w510:errorcluster, "Coefficients (µm)"=w509:sgl[], "Data Haso (dup)"=w508:T4)  [unwired: 3 in]
                              "Model Coefficients (µm) after" <- w509
                              n167 = Bundle By Name(cluster=T3 {"Filtre tilt X"=FALSE, "Filtre tilt Y"=FALSE, "Filtre courbure"=FALSE} ("Filtre"), "Filtre tilt X"="Filter x tilt", "Filtre tilt Y"="Filter y tilt", "Filtre courbure"="Curvature filter") -> (w532:T3)
                              n168 = call <vilib>:"DataHaso parameters.vi"("error in (no error)"=w510, "Data Haso"=w508) -> ("error out"=w542:errorcluster, "Parameters"=w521:T1, "Data Haso (dup)"=w543:T4)  [unwired: 3 in]
                              "after correction" <- w521
                              n169 = control-ref of="after correction"() -> (w526:refnum<vi>)
                              n170 = call "DataHaso filter tilt or curvature.vi"("error in (no error)"=w542, "Filter (default: all true)"=w532, "Data Haso"=w543) -> ("error out"=w540:errorcluster, "Data Haso (dup)"=w541:T4)  [unwired: 3 in]
                              n171 = call "DataHaso phase.vi"("error in (no error)"=w540, "Data Haso"=w541) -> ("error out"=w538:errorcluster, "Phase (µm)"=w539:i32, "Data Haso (dup)"=w525:T4)  [unwired: 3 in]
                              n172 = call "Formatter Intensity Graph.vi"("error in (no error)"=w538, "Intensity Graph"=w526, "Surface with pupil"=w539) -> ("error out"=w536:errorcluster, "Surface with pupil (dup)"=w537:i32)  [unwired: 2 in, 1 out]
                              n173 = call <vilib>:"Surface with pupil get stats.vi"("error in (no error)"=w536, "Surface Avec Pupille"=w537) -> ("error out"=w557:errorcluster, "PV"=w522:sgl, "RMS"=w523:dbl)  [unwired: 2 in, 1 out]
                              "RMS" <- w523
                              "PV" <- w522
                              n174 = Merge Errors(w557, w548) -> (w556:errorcluster)
                              n175 = Bundle By Name(cluster=T6 {"Target for tilt"=0, "Target for focus"=0, "Target for all other aberrations"=0} ("References"), "Target for tilt"=w506, "Target for focus"=w506) -> (w560:T6)
                              n176 = call "DataHaso ctor copie.vi"("error in (no error)"=w556, "DataHaso"=w525) -> ("error out"=w559:errorcluster, "new DataHaso"=w558:T4, "DataHaso (dup)"=w524:T4)  [unwired: 3 in]
                              n177 = call "Casao Compute target.vi"("error in (no error)"=w559, "Targets"=w560, "DataHaso"=w558, "Casao"=w549) -> ("error out"=w554:errorcluster, "DataHaso (dup)"=w528:T4, "Casao (dup)"=w555:T10)  [unwired: 1 out]
                              n178 = Bundle By Name(cluster=T5 {"Measurement"=0, "Target"=0, "Manual target"=0} ("Slopes"), "Measurement"=w524, "Target"=w528) -> (w553:T5)
                              n179 = call "Casao get correction commands.vi"("Casao"=w555, "Slopes"=w553, "error in (no error)"=w554) -> ("Casao (dup)"=w527:T10, "Commands"=w520:sgl[], "error out"=w500:errorcluster)  [unwired: 2 in, 2 out]
                              n180 = case shown="True" w503 {
                                tunnel: w500 -> [_ w567]
                                tunnel: w520 -> [_ w566]
                                tunnel: w507 -> [_ w565]
                                frame False {
                                }
                                frame True {
                                n181 = call "PhaseModul apply command.vi"("error in (no error)"=w567, "Commands in"=w566, "Mirror"=w565) -> ()  [unwired: 2 in, 3 out]
                                }
                              }
                            }
                            frame #4 {
                              n182 = call "DataHaso dtor.vi"("Data Haso"=w576) -> ()  [unwired: 6 in, 1 out]
                              n183 = case shown="Error" w570 {
                                tunnel: w569 -> [w577 _]
                                tunnel: [w577 w578] -> w568
                                frame No Error {
                                }
                                frame Error {
                                n184 = Initialize Array(0.0 ("element"), 52 ("dimension size")) -> (w578:dbl[])
                                }
                              }
                            }
                          }
                        }
                      }
                      frame #4 {
                        n185 = call "DataHaso dtor.vi"("Data Haso"=w586) -> ()  [unwired: 6 in, 1 out]
                        n186 = local read "Slice now"() -> (w591:dbl)
                        n187 = Cluster To Array(cluster=w597) -> (array=w596:sgl[])
                        n188 = Build Array (concatenate)(w598, w599, w596, w588) -> (w604:dbl[])
                        n189 = Number To Decimal String(number=w591) -> (decimal integer string=w601:string)  [unwired: 1 in]
                        n190 = Number To Decimal String(number=w591) -> (decimal integer string=w593:string)  [unwired: 1 in]
                        n191 = call "AO single value.vi"("data"=0.0, "physical channels"=tag "Dev1/ao4") -> ()  [unwired: 1 in, 1 out]
                        n192 = call "AO single value.vi"("data"=-5.0, "physical channels"=tag "Dev1/ao5") -> ()  [unwired: 1 in, 1 out]
                        n193 = local read "output path"() -> (w585:path)
                        n194 = Concatenate Strings("afterC_slice", w601, ".dat") -> (w584:string)
                        n195 = Concatenate Strings("command", w593, ".dat") -> (w582:string)
                        n196 = Build Path(base path=w585, name or relative path=w584) -> (appended path=w583:path)
                        n197 = Build Path(base path=w585, name or relative path=w582) -> (appended path=w581:path)
                        n198 = call-poly <vilib>:"Write To Spreadsheet File.vi"("transpose? (no:F)"=TRUE, "format (%.3f)"="%.6f", "1D data"=w604, "file path (dialog if empty)"=w583) -> ()  [unwired: 4 in, 1 out]
                        n199 = call-poly <vilib>:"Write To Spreadsheet File.vi"("transpose? (no:F)"=TRUE, "format (%.3f)"="%.6f", "1D data"=w587, "file path (dialog if empty)"=w581) -> ()  [unwired: 4 in, 1 out]
                      }
                      frame #5 {
                        n200 = local read "Average Frame #"() -> (w611:dbl)
                        n201 = for {
                          N: w611 -> [_]
                          n202 = local read "stop"() -> (w612:bool)
                          n203 = Not(x=w612) -> (.not. x?=w613:bool)
                          n204 = case shown="True" w613 {
                            frame False {
                            }
                            frame True {
                              n205 = flat-sequence {
                                frame #0 {
                                n206 = local read "Laser Power%(0-100)"() -> (w624:dbl)
                                n207 = local read "ImExp Time (s)"() -> (w623:dbl)
                                n208 = call "waveform gen.vi"("Boolean"=TRUE, "Exposure Time (s)"=w623, "Laser Power%(0-100)"=w624) -> ("waveform"=w621:waveform(dbl)[])
                                n209 = Index Array(array=w621, index=4) -> (element=w622:waveform(dbl))
                                n210 = call "AO triggle.vi"("physical channels"=tag "Dev1/ao0:4", "data"=w621, "waveform"=w622, "trig source"=tag "/Dev1/PFI0") -> ("task out"=w618:refnum<k21>, "error out"=w615:errorcluster)  [unwired: 1 in]
                                n211 = call "DO single value.vi"("error in"=w615, "data"=TRUE, "lines"=tag "Dev1/port0/line0") -> ("error out"=w614:errorcluster)
                                n212 = while {
                                tunnel: [w633] -> w627
                                tunnel: [w632] -> w626
                                tunnel: w618 -> [w630]
                                tunnel: w614 -> [w629]
                                stop <- w631 stop-if-true
                                n213 = call <vilib>:"DAQmx Is Task Done.vi"("task/channels in"=w630, "error in"=w629) -> ("task out"=w633:refnum<k21>, "task done?"=w631:bool, "error out"=w632:errorcluster)  [unwired: 11 in]
                                }
                                n214 = call <vilib>:"DAQmx Clear Task.vi"("task in"=w627, "error in"=w626) -> ()  [unwired: 13 in, 1 out]
                                }
                                frame #1 {
                                n215 = call "AO single value.vi"("data"=0.0, "physical channels"=tag "Dev1/ao4") -> ()  [unwired: 1 in, 1 out]
                                n216 = call "DO single value.vi"("data"=FALSE, "lines"=tag "Dev1/port0/line0") -> ()  [unwired: 1 in, 1 out]
                                }
                              }
                            }
                          }
                        }
                      }
                      frame #6 {
                        n217 = local read "Step size(um)"() -> (w644:dbl)
                        n218 = Multiply(x=w644, y=10.0) -> (x*y=w642:dbl)
                        n219 = Number To Decimal String(number=w642) -> (decimal integer string=w639:string)  [unwired: 1 in]
                        n220 = Concatenate Strings("movrel z=", w639) -> (w640:string)
                        n221 = call "WriteCmd.vi"("Command"=w640, "VISA resource name"=refnum<visa-resource-name> "COM1") -> ()  [unwired: 1 in, 1 out]
                      }
                      frame #7 {
                        n222 = Wait (ms)(milliseconds to wait=u32 50) -> ()  [unwired: 1 out]
                      }
                    }
                  }
                }
                n223 = call "AO single value.vi"("data"=0.0, "physical channels"=tag "Dev1/ao4") -> ()  [unwired: 1 in, 1 out]
              }
            }
            frame #2 {
              n224 = call "Casao dtor.vi"("Casao"=w646) -> ()  [unwired: 6 in, 1 out]
            }
          }
        }
      }
    }
    frame #2 {
      n225 = call "AO single value.vi"("data"=0.0, "physical channels"=tag "Dev1/ao4") -> ()  [unwired: 1 in, 1 out]
      n226 = call "DO single value.vi"("data"=FALSE, "lines"=tag "Dev1/port0/line1") -> ()  [unwired: 1 in, 1 out]
      n227 = call "DO single value.vi"("data"=FALSE, "lines"=tag "Dev1/port0/line0") -> ()  [unwired: 1 in, 1 out]
    }
  }
